vi "Global Vars.vi"() -> ()   [LabVIEW 2020]
uses:
  DMM/Typedefs/DMM Control Variable References.ctl
  Power Supply/Typedefs/PS Control Variable References.ctl
panel:
  in  "Amp Power Supply Controls 2":T1
  in  "Diode Power Supply Controls":T1
  in  "DMM 2 Controls":T3
  in  "DMM 1 Controls":T3
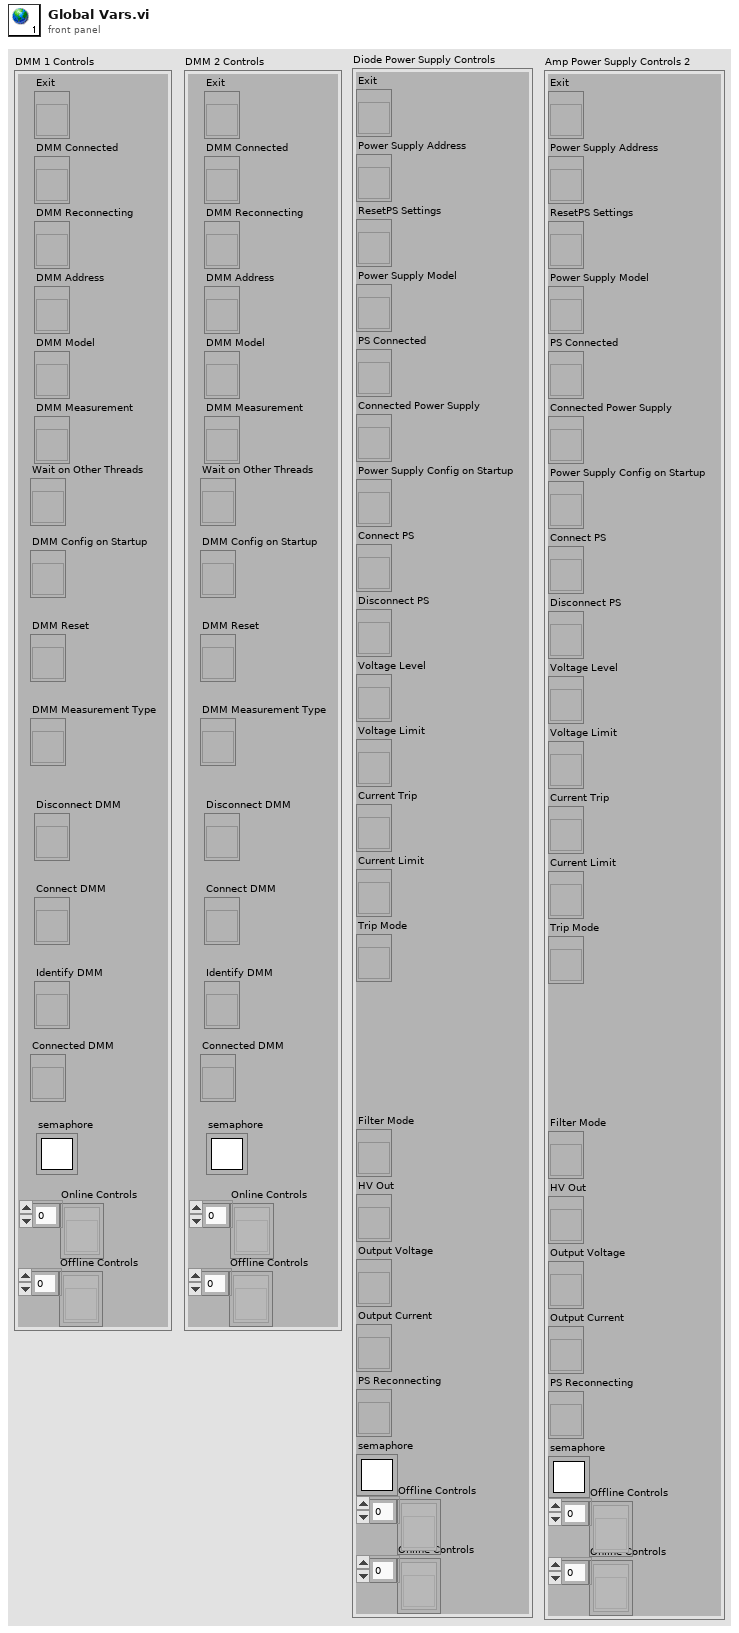
[diagram p1: front panel]
types:
  T1 = typedef "PS Control Variable References.ctl" = cluster{"Exit":refnum<vi>, "Power Supply Address":refnum<vi>, "ResetPS Settings":refnum<vi>, "Power Supply Model":refnum<vi>, "PS Connected":refnum<vi>, "Connected Power Supply":refnum<vi>, "Power Supply Config on Startup":refnum<vi>, "Connect PS":refnum<vi>, "Disconnect PS":refnum<vi>, "Voltage Level":refnum<vi>, "Voltage Limit":refnum<vi>, "Current Trip":refnum<vi>, "Current Limit":refnum<vi>, "Trip Mode":refnum<vi>, "Filter Mode":refnum<vi>, "HV Out":refnum<vi>, "Output Voltage":refnum<vi>, "Output Current":refnum<vi>, "PS Reconnecting":refnum<vi>, "semaphore":T2, "Offline Controls":refnum<vi>[], "Online Controls":refnum<vi>[]}
  T2 = typedef "Semaphore RefNum" = refnum<k1>
  T3 = typedef "DMM Control Variable References.ctl" = cluster{"Exit":refnum<vi>, "DMM Connected":refnum<vi>, "DMM Reconnecting":refnum<vi>, "DMM Address":refnum<vi>, "DMM Model":refnum<vi>, "DMM Measurement":refnum<vi>, "Wait on Other Threads":refnum<vi>, "DMM Reset":refnum<vi>, "DMM Config on Startup":refnum<vi>, "DMM Measurement Type":refnum<vi>, "Disconnect DMM":refnum<vi>, "Connect DMM":refnum<vi>, "Identify DMM":refnum<vi>, "Connected DMM":refnum<vi>, "semaphore":T2, "Online Controls":refnum<vi>[], "Offline Controls":refnum<vi>[]}
diagram:
